vi "Read Alarm Notifications.vi"(0 "VISA resource name":refnum<visa-resource-name>, 1 "Unit Address (1)":u8=1 min=1 max=254, 11 "error in (no error)":errorcluster) -> (4 "VISA resource name out":refnum<visa-resource-name>, 6 "New Alarm":bool, 15 "error out":errorcluster)   [LabVIEW 2010, in "Eurotherm 32xx Series.lvlib"]
doc: "This VI reads Alarm notification values."
uses:
  <instrlib>/Eurotherm 32xx Series/Eurotherm 32xx Series.lvlib
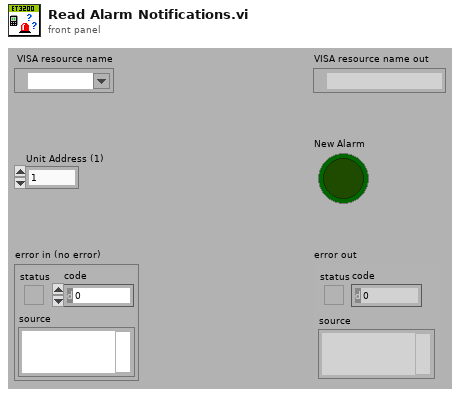
[diagram p1: front panel]
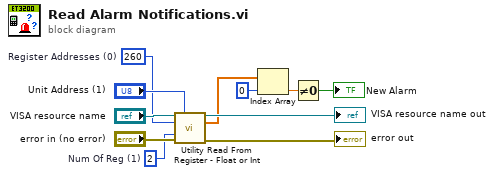
[diagram p0: block diagram]
diagram:
  w6 = u16 2  # Num Of Reg (1)
  w1 = u16 260  # Register Addresses (0)
  n1 = call <instrlib>:"Utility Read From Register - Float or Int.vi"("VISA resource name"="VISA resource name", "Unit Address (1)"="Unit Address (1)", "Register Address (0)"=w1, "Num Of Reg (1)"=w6, "error in (no error)"="error in (no error)") -> ("VISA resource name out"=→"VISA resource name out":refnum<visa-resource-name>, "Data"=w5:sgl[], "error out"=→"error out":errorcluster)  [unwired: 8 in]
  n2 = Index Array(array=w5, index=0) -> (element=w3:sgl)
  n3 = Not Equal To 0?(x=w3) -> (x != 0?=→"New Alarm":bool)
